vi "Configure Battery Stop Type.vi"(0 "VISA resource name":refnum<visa-resource-name>, 1 "Stop Type":u16(ring) items=["Voltage", "Current", "Capacity", "Time"], 2 "Level(V\\A\\Ah\\S)":dbl min=0.0, 3 "error in":errorcluster) -> (7 "VISA resource name out":refnum<visa-resource-name>, 10 "error out":errorcluster)   [LabVIEW 2018, in "IT-M3100.lvlib"]
doc: "This command to set the battery stop condition.s\n<b>Stop Type</b>\n0:Voltage:This command sets the cut off voltage.\n1:Current:This command sets the cut off current.\n2:Capacity:This command sets the cut off capacity.\n3:Time:This command sets the charging time.\n<b>Level(V\\A\\Ah\\S)</b>\n0-MAX"
uses:
  IT-M3100.lvlib
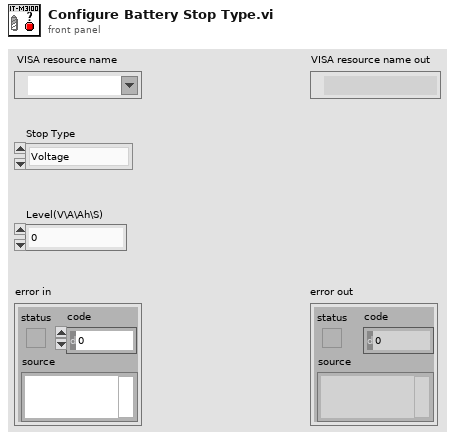
[diagram p1: front panel]
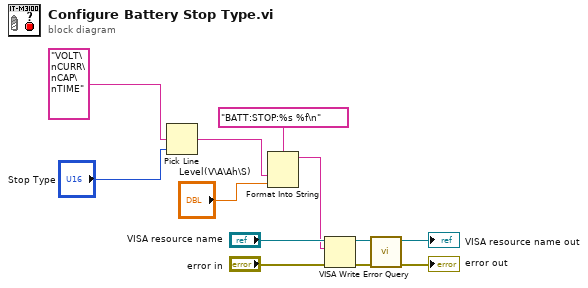
[diagram p0: block diagram]
diagram:
  n1 = Pick Line(multi-line string="VOLT\nCURR\nCAP\nTIME", line index="Stop Type") -> (output string=w2:string)  [unwired: 1 in]
  n2 = Format Into String(format string="BATT:STOP:%s %f\n", w2, "Level(V\\A\\Ah\\S)") -> (resulting string=w5:string)  [unwired: 2 in, 1 out]
  n3 = VISA Write(VISA resource name="VISA resource name", write buffer=w5, error in (no error)="error in") -> (VISA resource name out=w9:refnum<visa-resource-name>, error out=w10:errorcluster)  [unwired: 1 out]
  n4 = call "Error Query.vi"("error in"=w10, "VISA resource name"=w9) -> ("error out"=→"error out":errorcluster, "VISA resource name out"=→"VISA resource name out":refnum<visa-resource-name>)  [unwired: 6 in, 2 out]
